vi "Actuator module.vi"(8 "error in (no error)":errorcluster) -> (0 "error out":errorcluster)   [LabVIEW 2016]
uses:
  General/Controls/Queue modes.ctl
  General/Controls/States.ctl
  Controls/Actuator fgv modes.ctl
  General/Controls/staus modes.ctl
  Controls/Command cluster.ctl
  Controls/Command list.ctl
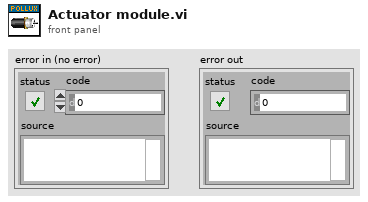
[diagram p1: front panel]
types:
  T1 = typedef "Queue modes.ctl" = enum16{"Initialise", "Destroy", "Get"}
  T2 = typedef "References.ctl" = cluster{"Tab Control":refnum<vi>, "Logo 1":refnum<vi>, "Logo 2":refnum<vi>, "Connect Actuator":refnum<vi>, "LIVE DATA":refnum<vi>, "Speed":refnum<vi>, "Home position":refnum<vi>, "Limit position":refnum<vi>, "Trigger":refnum<vi>, "Current position":refnum<vi>, "Connect Camera":refnum<vi>, "TEST DATA":refnum<vi>, "LIVE DATA Force":refnum<vi>, "Connect DAQ":refnum<vi>, "Initialised":refnum<vi>, "Test":refnum<vi>}
  T3 = typedef "Actuator fgv modes.ctl" = enum16{"Initalise", "COM", "Limit", "Speed", "Home", "Get"}
  T4 = typedef "staus modes.ctl" = enum16{"Status", "Testing", "Webcam", "DAQ", "Actuator", "Initialise"}
  T5 = typedef "Command cluster.ctl" = cluster{"Command":T6, "data":variant}
  T6 = typedef "Command list.ctl" = enum16{"", "£nabort", "getaxisno", "£getserialno", "£nidentify", "&&£setnlimit", "&£nm", "&£snv", "&£speed", "£np", "£ncal"}
  T7 = typedef "States.ctl" = enum16{"Initialise", "Actuator connection", "Get info", "Send command", "Load method", "Run method", "Save test", "Setup", "Shutdown"}
  T8 = typedef "State control cluster.ctl" = cluster{"State":T7, "Data":variant}
  T9 = typedef "Default settings.ctl" = cluster{"COM port":refnum<visa-resource-name>, "Home pos":dbl, "Speed":dbl, "Limit stop":dbl}
  T10 = typedef "UEs.ctl" = cluster{"Read position":refnum<user-event>, "Check home":refnum<user-event>, "Record":refnum<user-event>, "Abort controller":refnum<user-event>, "Remote test":refnum<user-event>, "Test setup":refnum<user-event>, "Conditional wait":refnum<user-event>, "Abort move":refnum<user-event>, "Wait done":refnum<user-event>, "Send trigger":refnum<user-event>, "Initalising":refnum<user-event>, "Initalisation complete":refnum<user-event>}
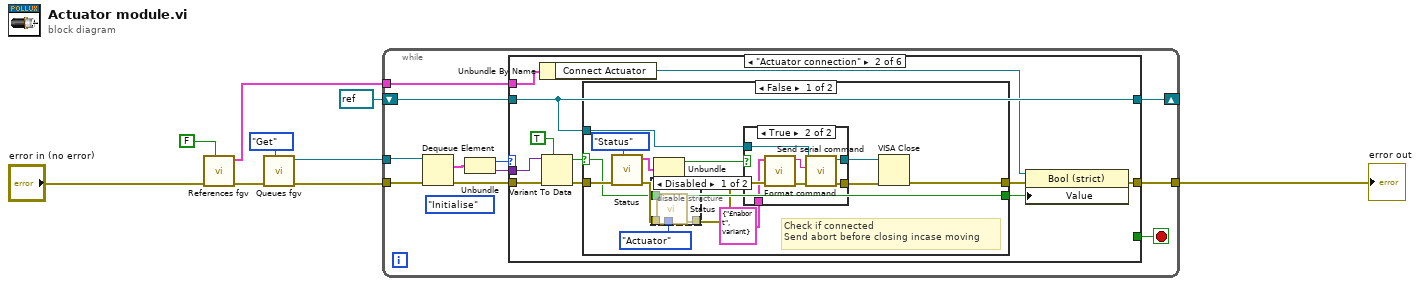
[diagram p0: block diagram]
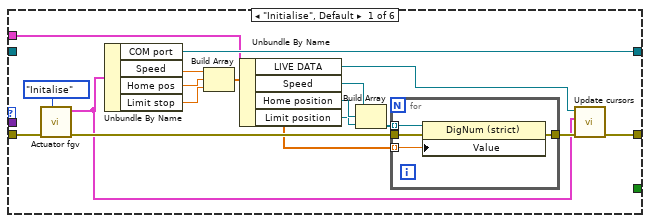
[diagram p2: hidden frame]
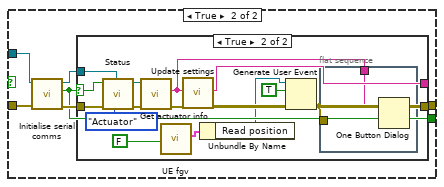
[diagram p5: hidden frame]
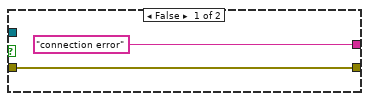
[diagram p6: hidden frame]
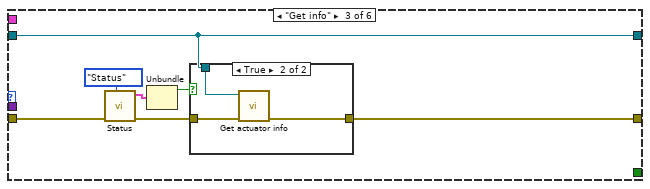
[diagram p7: hidden frame]
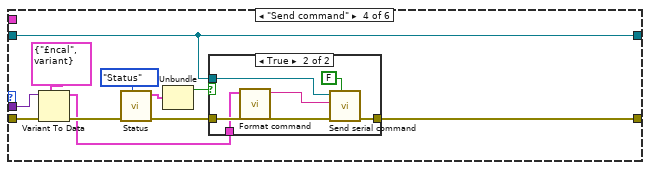
[diagram p9: hidden frame]
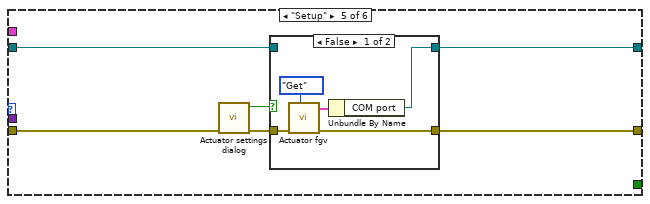
[diagram p11: hidden frame]
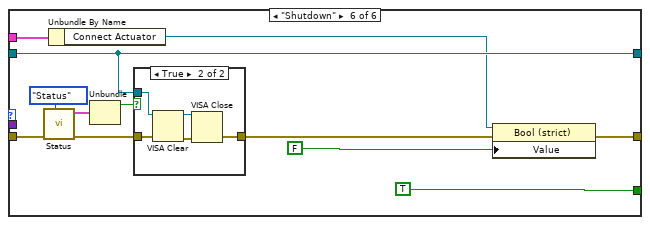
[diagram p13: hidden frame]
diagram:
  n1 = call "References fgv.vi"("Set?"=FALSE, "error in (no error)"="error in (no error)") -> ("error out"=w2:errorcluster, "Cluster"=w3:T2)  [unwired: 8 in]
  n2 = call "Queues fgv.vi"("Modes"=Queue_modes."Get", "error in (no error)"=w2) -> ("error in (no error) 2"=w8:errorcluster, "Ivium"=w7:refnum<queue>)  [unwired: 6 in, 2 out]
  n3 = while {
    tunnel: w7 -> [w20]
    tunnel: w8 -> [w19]
    tunnel: [w13] -> w6
    shift-right: [w11] -> _
    shift-left: refnum<visa-resource-name> refnum ("COM port") -> [w12]
    tunnel: w3 -> [w10]
    stop <- w14 stop-if-true
    (unwired) States."Initialise" ("State")
    n4 = Dequeue Element(queue=w20, error in (no error)=w19) -> (element=w18:T8, error out=w17:errorcluster)  [unwired: 1 in, 2 out]
    n5 = Unbundle(w18) -> ("State"=w16:T7, "Data"=w15:variant)
    n6 = case shown="\"Actuator connection\"" w16 {
      tunnel: w17 -> [w36 w50 w104 w116 w135 w151]
      tunnel: w15 -> [_ w52 _ w115 _ _]
      tunnel: [_ _ _ _ _ TRUE] -> w14
      tunnel: [w29 w49 w106 w121 w133 w153] -> w13
      tunnel: w12 -> [_ w48 w107 w122 w131 w146]
      tunnel: [w37 w48 w107 w122 w132 w146] -> w11
      tunnel: w10 -> [w25 w43 _ _ _ w144]
      frame "Initialise", Default {
        n7 = call "Actuator fgv.vi"("Enum"=Actuator_fgv_modes."Initalise", "error in (no error)"=w36) -> ("error out"=w32:errorcluster, "Cluster out"=w27:T9)  [unwired: 8 in]
        n8 = Unbundle By Name(w27) -> ("COM port"=w37:refnum<visa-resource-name>, "Speed"=w34:dbl, "Home pos"=w33:dbl, "Limit stop"=w26:dbl)
        n9 = Build Array(w34, w33, w26) -> (w30:dbl[])
        n10 = Unbundle By Name(w25) -> ("LIVE DATA"=w24:refnum<vi>, "Speed"=w23:refnum<vi>, "Home position"=w22:refnum<vi>, "Limit position"=w21:refnum<vi>)
        n11 = Build Array(w23, w22, w21) -> (w31:refnum<vi>[])
        n12 = for {
          tunnel: w32 -> [w41]
          tunnel: w31 -> [w40] mode=indexing
          tunnel: w30 -> [w39] mode=indexing
          tunnel: [w38] -> w28
          n13 = property class="DigNum (strict)"(reference=w40, error in=w41, "Value"=w39) -> (error out=w38:errorcluster)  [unwired: 1 out]
        }
        n14 = call "Update cursors.vi"("error in (no error)"=w28, "Cluster in"=w27, "LIVE DATA 3"=w24) -> ("error out"=w29:errorcluster)  [unwired: 8 in]
      }
      frame "Actuator connection" {
        n15 = Unbundle By Name(w43) -> ("Connect Actuator"=w42:refnum<vi>)
        n16 = Variant To Data(error in=w50, type=TRUE, Variant=w52) -> (data=w47:bool, error out=w46:errorcluster)
        n17 = case shown="False" w47 {
          selector: w47 -> [w54 _]
          tunnel: w48 -> [w58 w84]
          tunnel: [w54 w81] -> w44
          tunnel: w46 -> [w64 w80]
          tunnel: [w65 w79] -> w45
          frame False {
            # "Check if connected\nSend abort before closing incase moving"
            n18 = call "Status.vi"("Mode"=staus_modes."Status", "error in (no error)"=w64) -> ("error out"=w55:errorcluster, "Connections"=w62:cluster{"Data":bool, "Data":bool, "Data":bool})  [unwired: 7 in, 1 out]
            n19 = disable-structure shown="Disabled" {
              disable-tunnel: staus_modes."Actuator" ("Mode") -> [w69 _]
              disable-tunnel: w55 -> [w68 _]
              disable-tunnel: w54 -> [w67 _]
              disable-tunnel: [w66 _] -> w53
              frame Disabled {
                n20 = call "Status.vi"("Mode"=w69, "error in (no error)"=w68, "Data"=w67) -> ("error out"=w66:errorcluster)  [unwired: 6 in, 2 out]
              }
              frame Enabled {
              }
            }
            n21 = Unbundle(w62) -> ("Data"=w61:bool)  [unwired: 2 out]
            n22 = case shown="True" w61 {
              tunnel: w53 -> [w70 w78]
              tunnel: T5 {"Command"=enum."£nabort", "data"=variant} ("Cluster 2") -> [_ w77]
              tunnel: [w70 w75] -> w59
              tunnel: w58 -> [w71 w74]
              tunnel: [w71 w72] -> w57
              frame False {
              }
              frame True {
                n23 = call "Format command.vi"("error in (no error)"=w78, "Cluster"=w77) -> ("error out"=w76:errorcluster, "String"=w73:string)  [unwired: 8 in]
                n24 = call "Send serial command.vi"("error IO"=w76, "Send string"=w73, "VISA resource name out"=w74) -> ("error out"=w75:errorcluster, "VISA Out"=w72:refnum<visa-resource-name>)  [unwired: 6 in, 1 out]
              }
            }
            n25 = VISA Close(VISA resource name=w57, error in (no error)=w59) -> (error out=w65:errorcluster)
          }
          frame True {
            n26 = call "Initialise serial comms.vi"("error in (no error)"=w80, "VISA Refnum in"=w84) -> ("error out"=w83:errorcluster, "Connected?"=w81:bool, "VISA Refnum out"=w82:refnum<visa-resource-name>)  [unwired: 7 in]
            n27 = case shown="True" w81 {
              selector: w81 -> [_ w95]
              tunnel: w83 -> [w85 w97]
              tunnel: w82 -> [_ w99]
              tunnel: ["connection error" ("String") w87] -> _
              tunnel: [w85 w88] -> w79
              frame False {
              }
              frame True {
                n28 = call "Status.vi"("Mode"=staus_modes."Actuator", "error in (no error)"=w97, "Data"=w95) -> ("error out"=w96:errorcluster)  [unwired: 6 in, 2 out]
                n29 = call "Get actuator info.vi"("error in (no error)"=w96, "VISA Refnum in"=w99) -> ("error out"=w93:errorcluster, "String"=w87:string)  [unwired: 7 in, 1 out]
                n30 = call "UE fgv.vi"("Set?"=FALSE) -> ("UEs"=w90:T10)  [unwired: 8 in, 2 out]
                n31 = call "Update settings.vi"("error in (no error)"=w93) -> ("error out"=w92:errorcluster)  [unwired: 10 in]
                n32 = Unbundle By Name(w90) -> ("Read position"=w89:refnum<user-event>)
                n33 = Generate User Event(user event=w89, event data cluster=TRUE ("event data"), error in=w92) -> (error out=w88:errorcluster)  [unwired: 1 in, 1 out]
                n34 = flat-sequence {
                  tunnel: w88 -> [_]
                  tunnel: w87 -> [w100]
                  frame #0 {
                    n35 = One Button Dialog(message=w100) -> ()  [unwired: 1 in, 1 out]
                  }
                }
              }
            }
          }
        }
        n36 = property class="Bool (strict)"(reference=w42, error in=w45, "Value"=w44) -> (error out=w49:errorcluster)  [unwired: 1 out]
      }
      frame "Get info" {
        n37 = call "Status.vi"("Mode"=staus_modes."Status", "error in (no error)"=w104) -> ("error out"=w103:errorcluster, "Connections"=w105:cluster{"Data":bool, "Data":bool, "Data":bool})  [unwired: 7 in, 1 out]
        n38 = Unbundle(w105) -> ("Data"=w102:bool)  [unwired: 2 out]
        n39 = case shown="True" w102 {
          tunnel: w107 -> [_ w111]
          tunnel: [w108 w109] -> w106
          tunnel: w103 -> [w108 w110]
          frame False {
          }
          frame True {
            n40 = call "Get actuator info.vi"("error in (no error)"=w110, "VISA Refnum in"=w111) -> ("error out"=w109:errorcluster)  [unwired: 7 in, 2 out]
          }
        }
      }
      frame "Send command" {
        n41 = Variant To Data(error in=w116, type=T5 {"Command"=enum."£ncal", "data"=variant} ("Cluster"), Variant=w115) -> (data=w112:T5, error out=w113:errorcluster)
        n42 = call "Status.vi"("Mode"=staus_modes."Status", "error in (no error)"=w113) -> ("error out"=w119:errorcluster, "Connections"=w120:cluster{"Data":bool, "Data":bool, "Data":bool})  [unwired: 7 in, 1 out]
        n43 = Unbundle(w120) -> ("Data"=w118:bool)  [unwired: 2 out]
        n44 = case shown="True" w118 {
          tunnel: w122 -> [_ w127]
          tunnel: [w123 w129] -> w121
          tunnel: w119 -> [w123 w128]
          tunnel: w112 -> [_ w126]
          frame False {
          }
          frame True {
            n45 = call "Format command.vi"("Cluster"=w126) -> ("String"=w125:string)  [unwired: 9 in, 1 out]
            n46 = call "Send serial command.vi"("Read?"=FALSE, "error IO"=w128, "Send string"=w125, "VISA resource name out"=w127) -> ("error out"=w129:errorcluster)  [unwired: 5 in, 2 out]
          }
        }
      }
      frame "Setup" {
        n47 = call "Actuator settings dialog.vi"("error in (no error)"=w135) -> ("error out"=w134:errorcluster, "Cancelled?"=w130:bool)  [unwired: 9 in]
        n48 = case shown="False" w130 {
          tunnel: w134 -> [w140 w141]
          tunnel: [w139 w141] -> w133
          tunnel: [w136 w142] -> w132
          tunnel: w131 -> [_ w142]
          frame False {
            n49 = call "Actuator fgv.vi"("Enum"=Actuator_fgv_modes."Get", "error in (no error)"=w140) -> ("error out"=w139:errorcluster, "Cluster out"=w137:T9)  [unwired: 8 in]
            n50 = Unbundle By Name(w137) -> ("COM port"=w136:refnum<visa-resource-name>)
          }
          frame True {
          }
        }
      }
      frame "Shutdown" {
        n51 = call "Status.vi"("Mode"=staus_modes."Status", "error in (no error)"=w151) -> ("error out"=w147:errorcluster, "Connections"=w149:cluster{"Data":bool, "Data":bool, "Data":bool})  [unwired: 7 in, 1 out]
        n52 = Unbundle By Name(w144) -> ("Connect Actuator"=w143:refnum<vi>)
        n53 = Unbundle(w149) -> ("Data"=w148:bool)  [unwired: 2 out]
        n54 = case shown="True" w148 {
          tunnel: w147 -> [w155 w159]
          tunnel: w146 -> [_ w156]
          tunnel: [w155 w160] -> w145
          frame False {
          }
          frame True {
            n55 = VISA Clear(VISA resource name=w156, error in (no error)=w159) -> (VISA resource name out=w157:refnum<visa-resource-name>, error out=w158:errorcluster)
            n56 = VISA Close(VISA resource name=w157, error in (no error)=w158) -> (error out=w160:errorcluster)
          }
        }
        n57 = property class="Bool (strict)"(reference=w143, error in=w145, "Value"=FALSE) -> (error out=w153:errorcluster)  [unwired: 1 out]
      }
    }
  }
  "error out" <- w6
